vi "send_command.vi"(8 "error in (no error)":errorcluster, 10 "command":string, 11 "connection ID":refnum<k5>) -> (0 "error out":errorcluster, 2 "response":string, 3 "connection ID out":refnum<k5>)   [LabVIEW 2024]
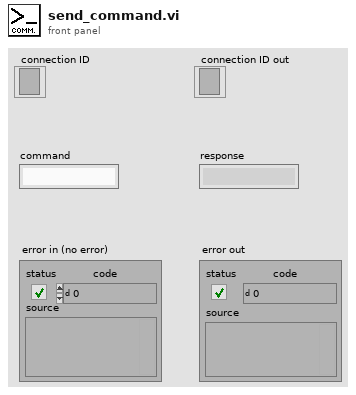
[diagram p1: front panel]
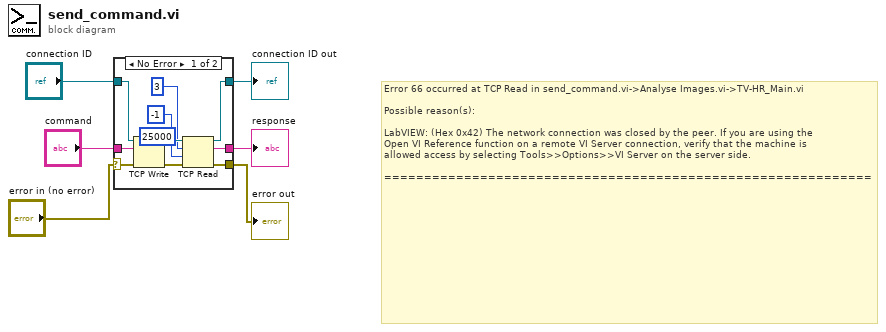
[diagram p0: block diagram]
diagram:
  # "Error 66 occurred at TCP Read in send_command.vi->Analyse Images.vi->TV-HR_Main.vi\n\nPossible reason(s):\n\nLabVIEW: (Hex 0x42) The network connection was closed by the peer. If you are using the \nOpen VI Reference function on a remote VI Server connection, verify that the machine is \nallowed access by selecting Tools>>Options>>VI Server on the server side.\n\n============================================================="
  n1 = case shown="No Error" "error in (no error)" {
    selector: "error in (no error)" -> [w13 w19]
    tunnel: [w12 w19] -> w5
    tunnel: "connection ID" -> [w11 w18]
    tunnel: [w10 w18] -> w3
    tunnel: "command" -> [w9 w17]
    tunnel: [w8 w17] -> w1
    frame No Error {
      (unwired) 25000 ("timeout ms (25000)")
      n2 = TCP Write(connection ID=w11, data in=w9, error in (no error)=w13) -> (connection ID out=w16:refnum<k5>, error out=w14:errorcluster)  [unwired: 1 in, 1 out]
      n3 = TCP Read(connection ID=w16, bytes to read=3, error in (no error)=w14, 9:-1 ("timeout ms (25000)")) -> (connection ID out=w10:refnum<k5>, data out=w8:string, error out=w12:errorcluster)  [unwired: 1 in]
    }
    frame Error {
    }
  }
  "error out" <- w5
  "connection ID out" <- w3
  "response" <- w1
